vi "Event Handler.vi"(8 "error in (no error)":errorcluster, 10 "Stop Event Handler":refnum<user-event>, 11 "QPicture in":refnum<class "QPicture.lvclass">) -> (0 "error out":errorcluster)   [LabVIEW 2019, in "QPicture.lvclass"]
doc: "The <b>Event Handler VI</b> is a dynamic dispatch VI that should be overwritten if events are needed to create the enhanced QControl. \n\nBy inheriting from the main Control.lvclass the overwritten <b>Event Handler VI</b> will be launched asynchronously in the initialization of the QControl.\n<b> </b> <b> </b>\n©2016 Q Software Innovations, LLC (QSI)\nwritten by Quentin Alldredge\nproduced in LabVIEW 2015\n\nsupport@qsoftwareinnovations.com\nwww.qsoftwareinnovations.com\n\nAll rights reserved.\n\nRedistribution and use in source and binary forms, with or without modification, are permitted provided that the following conditions are met:\n\n * Redistributions of source code must retain the above copyright notice, this list of conditions and the following disclaimer.\n * Redistributions in binary form must reproduce the above copyright notice, this list of conditions and the following disclaimer in the documentation and/or other materials provided with the distribution.\n * Neither the name of Q Software Innovations, LLC. nor the names of its contributors may be used to endorse or promote products derived from this software without specific prior written permission.\n\nTHIS SOFTWARE IS PROVIDED BY THE COPYRIGHT HOLDERS AND CONTRIBUTORS \"AS IS\" AND ANY EXPRESS OR IMPLIED WARRANTIES, INCLUDING, BUT NOT LIMITED TO, THE IMPLIED WARRANTIES OF MERCHANTABILITY AND FITNESS FOR A PARTICULAR PURPOSE ARE DISCLAIMED. IN NO EVENT SHALL THE COPYRIGHT OWNER OR CONTRIBUTORS BE LIABLE FOR ANY DIRECT, INDIRECT, INCIDENTAL, SPECIAL, EXEMPLARY, OR CONSEQUENTIAL DAMAGES (INCLUDING, BUT NOT LIMITED TO, PROCUREMENT OF SUBSTITUTE GOODS OR SERVICES; LOSS OF USE, DATA, OR PROFITS; OR BUSINESS INTERRUPTION) HOWEVER CAUSED AND ON ANY THEORY OF LIABILITY, WHETHER IN CONTRACT, STRICT LIABILITY, OR TORT (INCLUDING NEGLIGENCE OR OTHERWISE) ARISING IN ANY WAY OUT OF THE USE OF THIS SOFTWARE, EVEN IF ADVISED OF THE POSSIBILITY OF SUCH DAMAGE."
uses:
  QPicture.lvclass
  QPicture.lvclass/QPicture.ctl
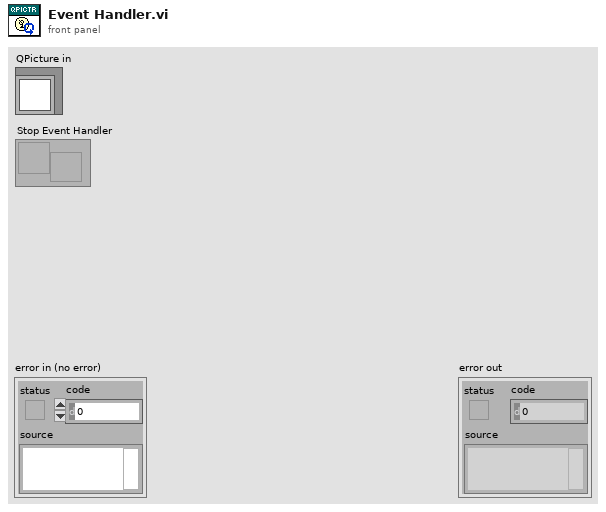
[diagram p1: front panel]
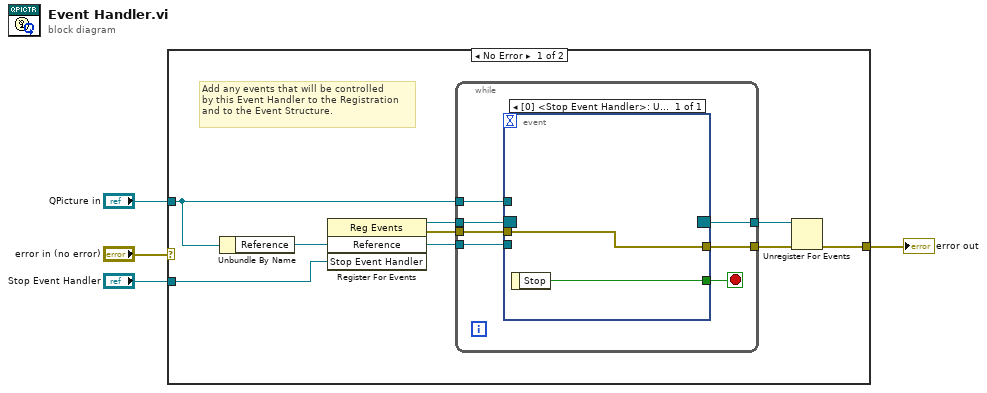
[diagram p0: block diagram]
diagram:
  n1 = case shown="No Error" "error in (no error)" {
    selector: "error in (no error)" -> [_ w22]
    tunnel: [w9 w22] -> w3
    tunnel: "QPicture in" -> [w7 _]
    tunnel: "Stop Event Handler" -> [w5 _]
    frame No Error {
      # "Add any events that will be controlled\nby this Event Handler to the Registration\nand to the Event Structure."
      n2 = Unbundle By Name(w7) -> ("Reference"=w6:refnum<vi>)
      n3 = register-events(w6, w5) -> (reference out=w12:refnum<event-registration>, error out=w11:errorcluster)  [unwired: 2 in]
      n4 = while {
        tunnel: w12 -> [w19]
        tunnel: w11 -> [w17]
        tunnel: [w16] -> w10
        tunnel: [w14] -> w8
        tunnel: w6 -> [w13]
        tunnel: w7 -> [w18]
        stop <- w15 stop-if-true
        n5 = event shown="[0] <Stop Event Handler>: User Event" {
          selector: w19 -> [_]
          dyn-events: [_] -> w14
          timeout: _ -> [_]
          tunnel: w18 -> [_]
          tunnel: w17 -> [w21]
          tunnel: [w21] -> w16
          tunnel: [w20] -> w15
          tunnel: w13 -> [_]
          event User Event {
            n6 = event-data() -> ("Stop"=w20:bool)  [unwired: 1 in]
          }
        }
      }
      n7 = Unregister For Events(event registration refnum=w8, error in=w10) -> (error out=w9:errorcluster)
    }
    frame Error {
    }
  }
  "error out" <- w3
